vi "Window Bounds Convert To Size.vi"(1 "Window Bounds":T2) -> (0 "Window Size":T1)   [LabVIEW 2015]
uses:
  <vilib>/Utility/miscctls.llb/LVRectTypeDef.ctl
  <vilib>/Utility/miscctls.llb/LVPointTypeDef.ctl
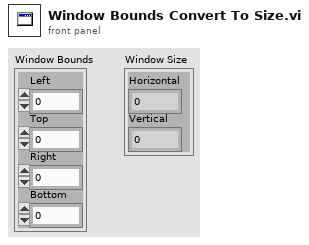
[diagram p1: front panel]
types:
  T1 = typedef "LVPointTypeDef.ctl" = cluster{"Horizontal":i16, "Vertical":i16}
  T2 = typedef "LVRectTypeDef.ctl" = cluster{"Left":i16, "Top":i16, "Right":i16, "Bottom":i16}
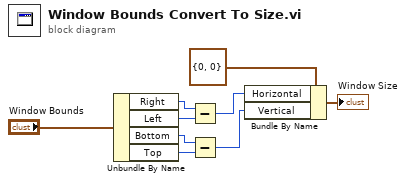
[diagram p0: block diagram]
diagram:
  n1 = Unbundle By Name("Window Bounds") -> ("Right"=w8:i16, "Left"=w7:i16, "Bottom"=w4:i16, "Top"=w3:i16)
  n2 = Subtract(x=w8, y=w7) -> (x-y=w5:i16)
  n3 = Subtract(x=w4, y=w3) -> (x-y=w2:i16)
  n4 = Bundle By Name(cluster=T1 {"Horizontal"=0, "Vertical"=0} ("Window Size"), "Horizontal"=w5, "Vertical"=w2) -> (→"Window Size":T1)
